vi "Load Rich Text Notebook.vi"(6 "Backup?":bool, 8 "Error In":errorcluster, 10 "File Path Control":path, 11 ".NET Refnum in":refnum<k24>) -> (0 "Error Out":errorcluster, 1 "cancelled":bool, 2 "File Path out":path, 3 ".NET Refnum out":refnum<k24>, 4 "RTF content":string)   [LabVIEW 2021, in "Notebook.lvlib"]
uses:
  Notebook.lvlib
  System.Windows.Forms
  Notebook Parameters List.ctl
  Variant/Variant to Data/Variant to Boolean.vi
  Variant/Variant to Data/Variant to Data.lvlib
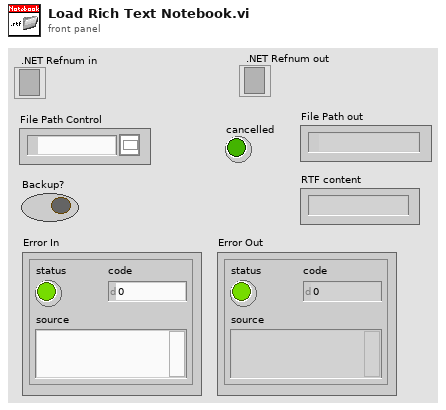
[diagram p1: front panel]
types:
  T1 = typedef "Notebook.lvlib/Notebook Parameters List.ctl" = enum16{"First Opening?", "Saved Notebook?", "Saved Notebook Path", "Beep on Error?"}
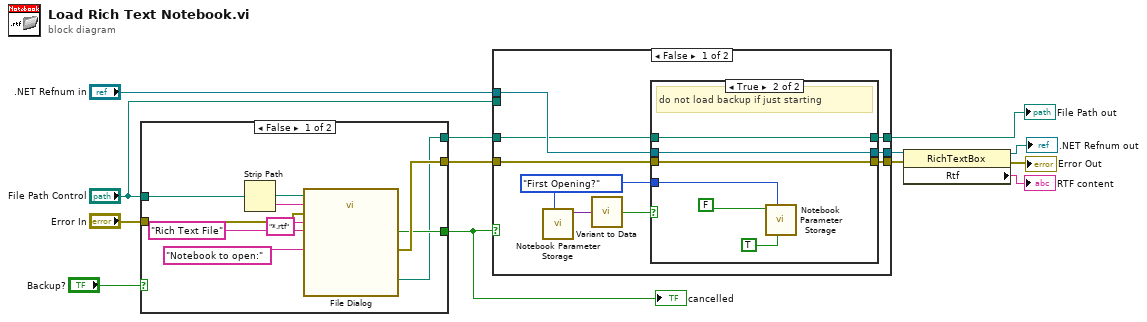
[diagram p0: block diagram]
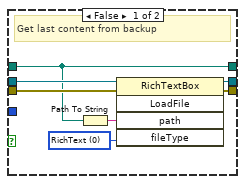
[diagram p3: hidden frame]
diagram:
  n1 = case shown="False" "Backup?" {
    tunnel: [w23 w24] -> w12
    tunnel: "Error In" -> [w22 w24]
    tunnel: [w16 _] -> w10
    tunnel: [w15 w25] -> w9
    tunnel: "File Path Control" -> [w14 w25]
    frame False {
      n2 = Strip Path(path=w14) -> (stripped path=w20:path, name=w19:string)
      n3 = call "File Dialog"("start path"=w20, "prompt"="Notebook to open:", "default name"=w19, "error in"=w22, "pattern (all files)"="*.rtf" ("pattern label"), "pattern label"="Rich Text File") -> ("selected path"=w15:path, "cancelled"=w16:bool, "error out"=w23:errorcluster)  [unwired: 6 in, 1 out]
    }
    frame True {
    }
  }
  "cancelled" <- w10
  n4 = case shown="False" w10 {
    tunnel: ".NET Refnum in" -> [w34 w48]
    tunnel: w12 -> [w33 w50]
    tunnel: [w31 w50] -> w6
    tunnel: w9 -> [w30 _]
    tunnel: [w29 w49] -> w8
    tunnel: "File Path Control" -> [_ w49]
    tunnel: [w32 w48] -> w7
    frame False {
      w28 = Notebook_Parameters_List."First Opening?" ("Notebook Parameter List")
      n5 = call "Notebook Parameter Storage.vi"("Notebook Parameter List"=w28) -> ("Data out"=w27:variant)  [unwired: 9 in, 1 out]
      n6 = call-poly "Variant to Data.vi"("Variant"=w27) -> ("Value"=w26:bool)  [unwired: 8 in]
      n7 = case shown="True" w26 {
        tunnel: w34 -> [w41 w46]
        tunnel: w33 -> [w40 w47]
        tunnel: [w38 w46] -> w32
        tunnel: [w37 w47] -> w31
        tunnel: w30 -> [w35 w45]
        tunnel: [w35 w45] -> w29
        tunnel: w28 -> [_ w42]
        frame False {
          w39 = 0 items=["RichText", "PlainText", "RichNoOleObjs", "TextTextOleObjs", "UnicodePlainText"] ("fileType")
          # "Get last content from backup"
          n8 = Path To String(path=w35) -> (string=w36:string)
          n9 = invoke class="RichTextBox" method="LoadFile"(reference=w41, error in=w40, "path"=w36, "fileType"=w39) -> (reference out=w38:refnum<k24>, error out=w37:errorcluster)  [unwired: 1 in, 3 out]
        }
        frame True {
          # "do not load backup if just starting"
          n10 = call "Notebook Parameter Storage.vi"("Get(F)/Set"=TRUE, "Notebook Parameter List"=w42, "Data in"=FALSE ("First opening?")) -> ()  [unwired: 7 in, 2 out]
        }
      }
    }
    frame True {
    }
  }
  "File Path out" <- w8
  n11 = property class="RichTextBox"(reference=w7, error in=w6) -> (reference out=→".NET Refnum out":refnum<k24>, error out=→"Error Out":errorcluster, "Rtf"=→"RTF content":string)
